vi "TypeConv_Register Existing Opaque Structs.vi"(6 "Projection Ref Map":variant, 9 "Classes":T1[](array[typedef]), 11 "Owning LVLib":refnum<vi>) -> ()   [LabVIEW 2013]
uses:
  Data Structures/JSON/Class.ctl
  Data Structures/JSON/Enum.ctl
  Data Structures/JSON/Enum Value.ctl
  Data Structures/JSON/Method.ctl
  Data Structures/JSON/Param.ctl
  Data Structures/JSON/Property.ctl
  Category.ctl
  Action.ctl
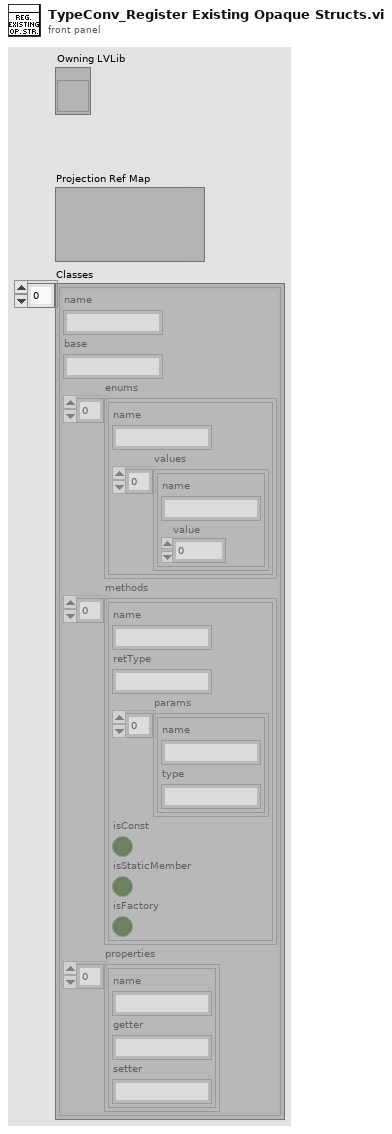
[diagram p1: front panel]
types:
  T1 = typedef "Class.ctl" = cluster{"name":string, "base":string, "enums":T2[], "methods":T4[], "properties":T6[]}
  T2 = typedef "Enum.ctl" = cluster{"name":string, "values":T3[]}
  T3 = typedef "Enum Value.ctl" = cluster{"name":string, "value":i32}
  T4 = typedef "Method.ctl" = cluster{"name":string, "retType":string, "params":T5[], "isConst":bool, "isStaticMember":bool, "isFactory":bool}
  T5 = typedef "Param.ctl" = cluster{"name":string, "type":string}
  T6 = typedef "Property.ctl" = cluster{"name":string, "getter":string, "setter":string}
  T7 = typedef "Category.ctl" = enum16{"Invalid", "Void", "Boolean", "Numeric", "Enum", "SimpleStruct", "OpaqueStruct", "SimpleIdentity", "QObject", "SimpleContainer", "FullArray"}
  T8 = typedef "Action.ctl" = enum16{"Register Type", "Obtain Writer"}
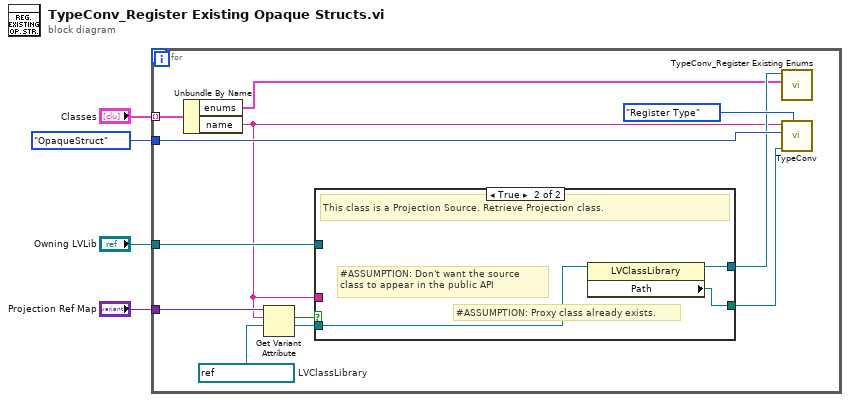
[diagram p0: block diagram]
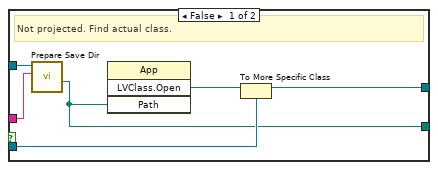
[diagram p2: hidden frame]
diagram:
  n1 = for {
    tunnel: "Classes" -> [w14] mode=indexing
    tunnel: "Projection Ref Map" -> [w13]
    tunnel: Category."OpaqueStruct" ("Category") -> [w9]
    tunnel: "Owning LVLib" -> [w16]
    w11 = refnum<vi> refnum  # LVClassLibrary
    n2 = Unbundle By Name(w14) -> ("enums"=w6:T2[], "name"=w5:string)
    n3 = Get Variant Attribute(Variant=w13, name=w5, default value (empty Variant)=w11) -> (found=w12:bool, value=w10:refnum<vi>)  [unwired: 1 in, 2 out]
    n4 = case shown="True" w12 {
      tunnel: w16 -> [w22 _]
      tunnel: w5 -> [w21 _]
      tunnel: [w20 w24] -> w7
      tunnel: w10 -> [w19 w25]
      tunnel: [w18 w23] -> w8
      frame False {
        # "Not projected. Find actual class."
        n5 = call "Prepare Save Dir.vi"("Entity Name"=w21, "Owning LVLib"=w22) -> ("Entity Path"=w18:path)  [unwired: 8 in, 1 out]
        n6 = invoke class="App" method="LVClass.Open"("Path"=w18) -> ("LVClass.Open"=w17:refnum<vi>)  [unwired: 3 in, 3 out]
        n7 = To More Specific Class(target class=w19, reference=w17) -> (specific class reference=w20:refnum<vi>)  [unwired: 1 in, 1 out]
      }
      frame True {
        # "#ASSUMPTION: Don't want the source\nclass to appear in the public API"
        # "#ASSUMPTION: Proxy class already exists."
        # "This class is a Projection Source. Retrieve Projection class."
        n8 = property class="LVClassLibrary"(reference=w25) -> (reference out=w24:refnum<vi>, "Path"=w23:path)  [unwired: 1 in, 1 out]
      }
    }
    n9 = call "TypeConv_Register Existing Enums.vi"("Enums"=w6, "Owning Lib"=w7) -> ()  [unwired: 9 in, 1 out]
    n10 = call "TypeConv.vi"("Action"=Action."Register Type", "Type Path [Enum, SimpleStruct, OpaqueStruct]"=w8, "Category"=w9, "Type Name"=w5) -> ()  [unwired: 7 in, 1 out]
  }
